vi "Query Octree with sphere.vi"(2 "Octree node array":T2[](array[typedef]), 3 "Sphere":T1) -> (0 "Stack error":errorcluster, 1 "Indices of possible triangles":i32[](array[numeric]))   [LabVIEW 2014]
uses:
  Typedefs/TreeNodeBox.ctl
  Typedefs/Quad.ctl
  Typedefs/Sphere.ctl
panel:
  out "Stack history":i32(graph)
  # "PN 18/01/2015"
  # "Vertices"
  # "Edges"
  # "Unit normal"
  # "Edge unit normals"
  # "Vertices"
  # "Edges"
  # "Unit normal"
  # "Edge unit normals"
  # "Vertices"
  # "Edges"
  # "Unit normal"
  # "Edge unit normals"
  # "Vertices"
  # "Edges"
  # "Unit normal"
  # "Edge unit normals"
  # "Vertices"
  # "Edges"
  # "Unit normal"
  # "Edge unit normals"
  # "Vertices"
  # "Edges"
  # "Unit normal"
  # "Edge unit normals"
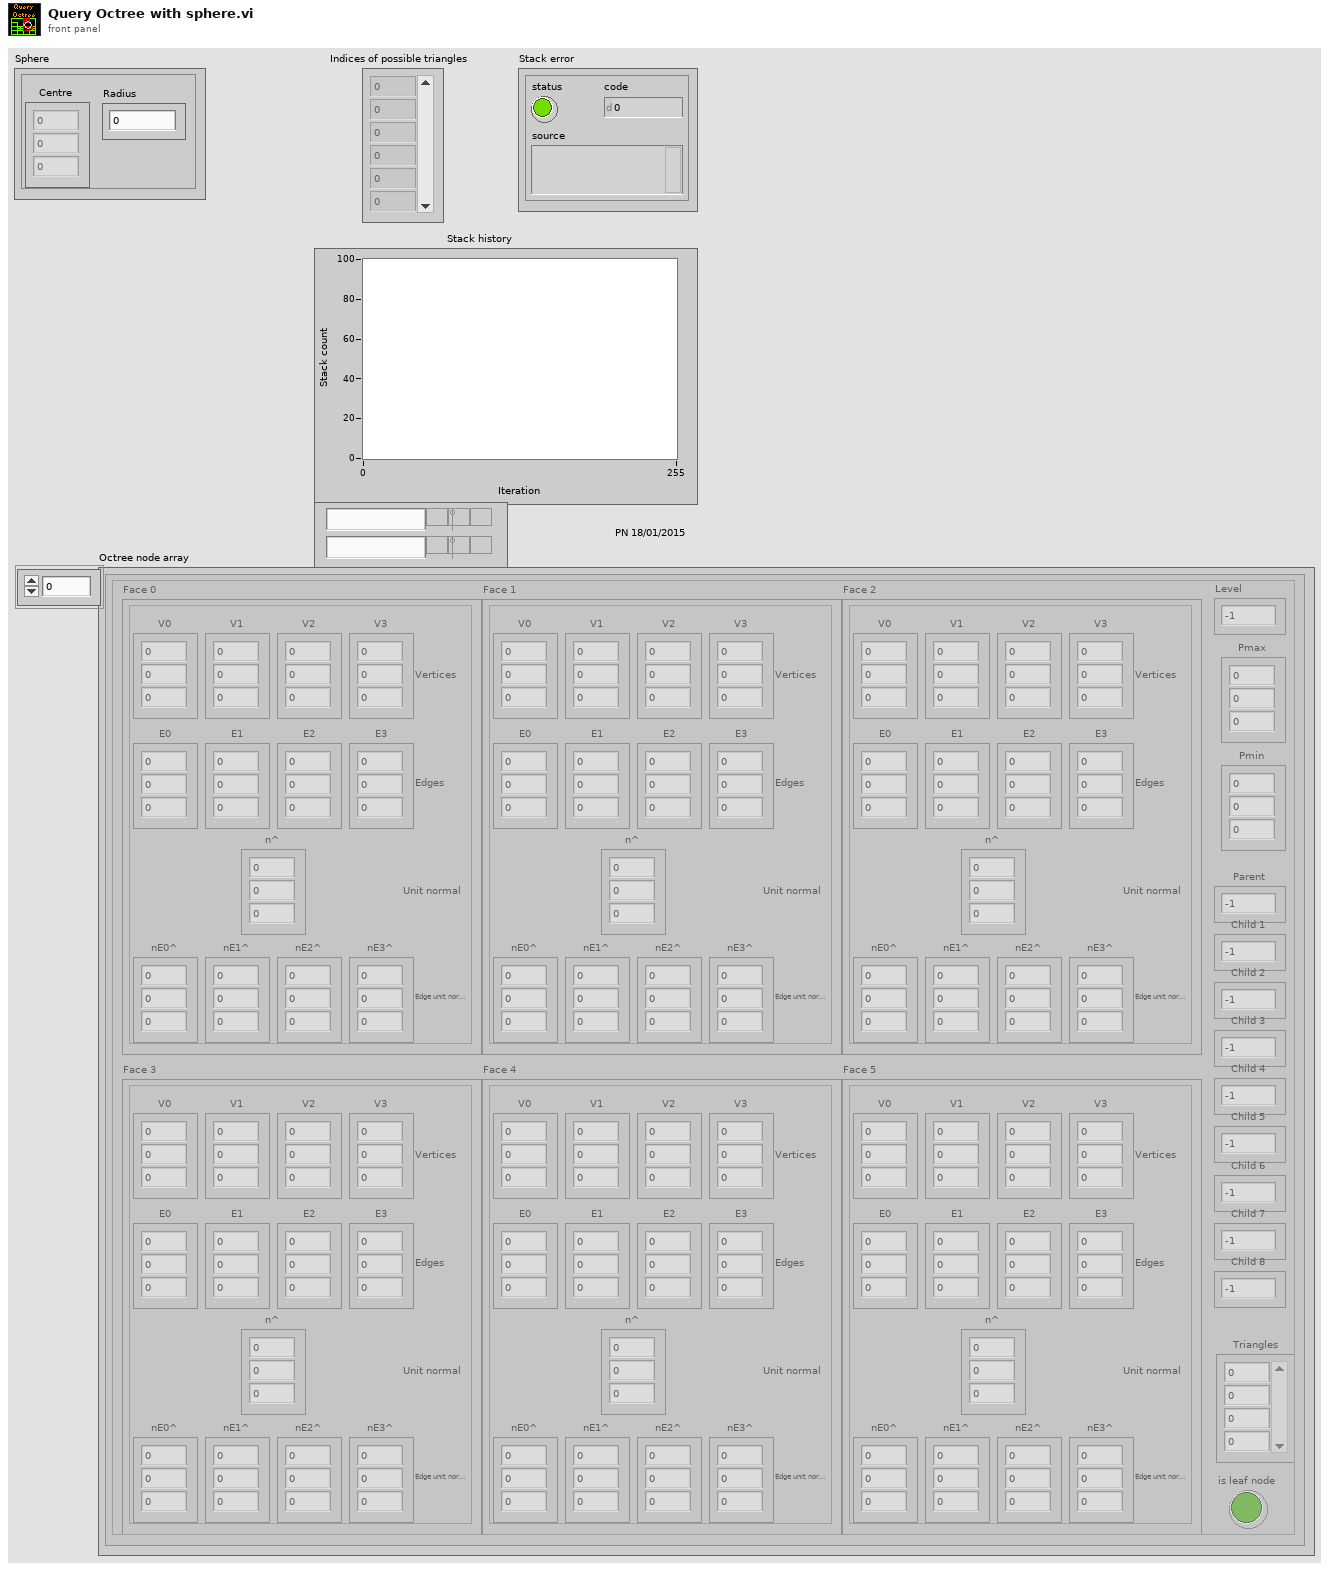
[diagram p1: front panel]
types:
  T1 = typedef "Sphere.ctl" = cluster{"Centre":sgl[], "Radius":sgl}
  T2 = typedef "TreeNodeBox.ctl" = cluster{"Face 0":T3, "Face 1":T3, "Face 2":T3, "Face 3":T3, "Face 4":T3, "Face 5":T3, "Level":i32, "Pmax":sgl[], "Pmin":sgl[], "Parent":i32, "Child 1":i32, "Child 2":i32, "Child 3":i32, "Child 4":i32, "Child 5":i32, "Child 6":i32, "Child 7":i32, "Child 8":i32, "Triangles":i32[], "is leaf node":bool}
  T3 = typedef "Quad.ctl" = cluster{"V0":sgl[], "V1":sgl[], "V2":sgl[], "V3":sgl[], "E0":sgl[], "E1":sgl[], "E2":sgl[], "E3":sgl[], "n^":sgl[], "nE0^":sgl[], "nE1^":sgl[], "nE2^":sgl[], "nE3^":sgl[]}
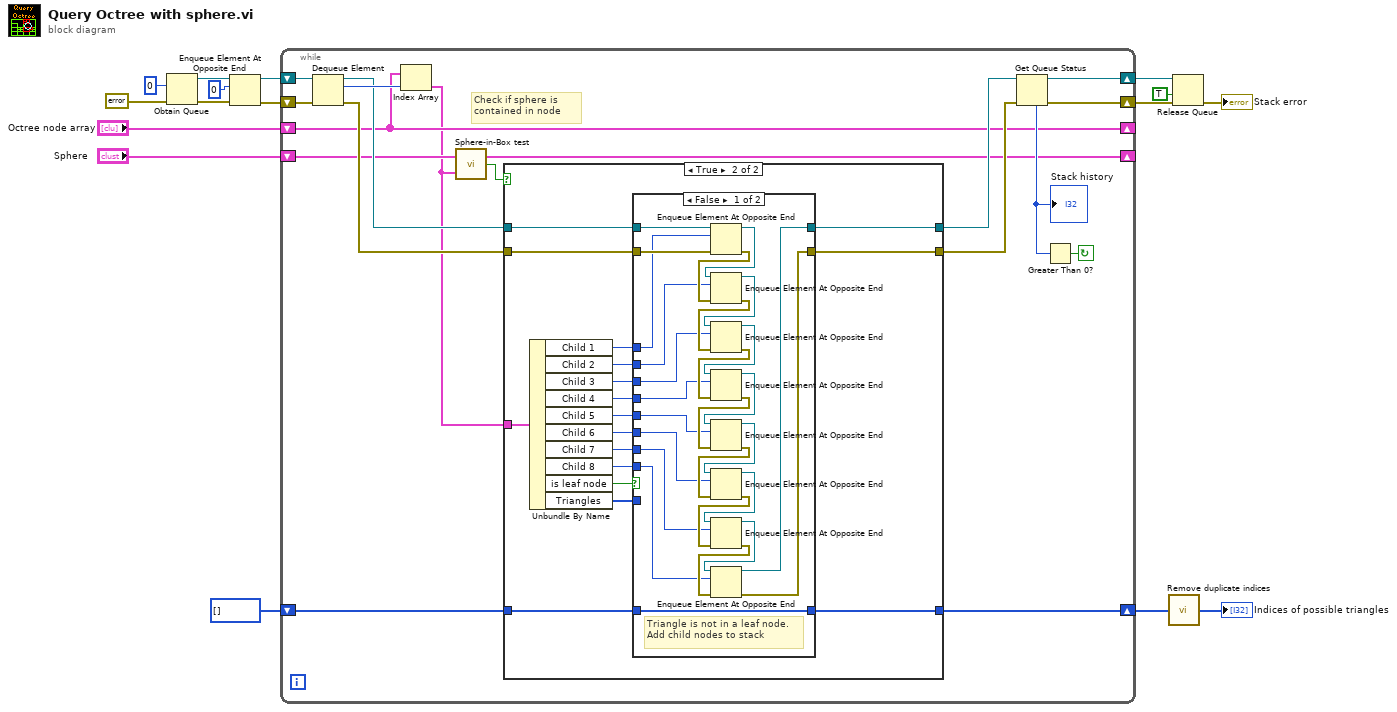
[diagram p0: block diagram]
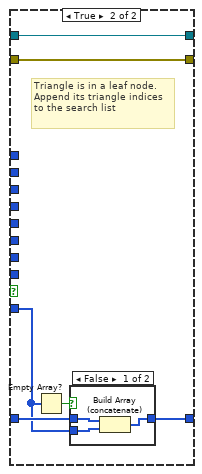
[diagram p3: hidden frame]
diagram:
  n1 = Obtain Queue(element data type=0, error in (no error)=errorcluster {"status"=FALSE, "code"=0, "source"=""}) -> (queue out=w15:refnum<queue>, error out=w14:errorcluster)  [unwired: 3 in, 1 out]
  n2 = Enqueue Element At Opposite End(queue=w15, element=0, error in (no error)=w14) -> (queue out=w13:refnum<queue>, error out=w12:errorcluster)  [unwired: 1 in, 1 out]
  n3 = while {
    shift-right: [w28] -> w11
    shift-left: w13 -> [w33]
    shift-right: [w30] -> w10
    shift-left: w12 -> [w32]
    shift-right: [w21] -> _
    shift-left: "Sphere" -> [w21]
    shift-right: [w20] -> _
    shift-left: "Octree node array" -> [w20]
    shift-right: [w17] -> w3
    shift-left: i32[] [] -> [w18]
    stop <- w31 continue-if-true
    # "Check if sphere is contained in node"
    n4 = Dequeue Element(queue=w33, error in (no error)=w32) -> (queue out=w27:refnum<queue>, element=w29:i32, error out=w26:errorcluster)  [unwired: 1 in, 1 out]
    n5 = Index Array(array=w20, index=w29) -> (element=w19:T2)
    n6 = call "Sphere-in-Box test.vi"("Box"=w19, "Sphere"=w21) -> ("Sphere is inside box"=w22:bool)
    n7 = case shown="True" w22 {
      tunnel: w27 -> [w35 w42]
      tunnel: [w35 w38] -> w25
      tunnel: [w36 w37] -> w24
      tunnel: w26 -> [w36 w41]
      tunnel: w19 -> [_ w53]
      tunnel: w18 -> [w34 w52]
      tunnel: [w34 w51] -> w17
      frame False {
        # "Triangle is not contained in node, continue"
      }
      frame True {
        n8 = Unbundle By Name(w53) -> ("Child 1"=w50:i32, "Child 2"=w49:i32, "Child 3"=w48:i32, "Child 4"=w47:i32, "Child 5"=w46:i32, "Child 6"=w45:i32, "Child 7"=w44:i32, "Child 8"=w43:i32, "is leaf node"=w40:bool, "Triangles"=w39:i32[])
        n9 = case shown="False" w40 {
          tunnel: w52 -> [w54 w85]
          tunnel: [w54 w84] -> w51
          tunnel: w50 -> [w64 _]
          tunnel: w49 -> [w63 _]
          tunnel: w48 -> [w62 _]
          tunnel: w47 -> [w61 _]
          tunnel: w46 -> [w60 _]
          tunnel: w45 -> [w59 _]
          tunnel: w44 -> [w58 _]
          tunnel: w43 -> [w57 _]
          tunnel: w39 -> [_ w83]
          tunnel: w42 -> [w66 w81]
          tunnel: w41 -> [w65 w82]
          tunnel: [w56 w81] -> w38
          tunnel: [w55 w82] -> w37
          frame False {
            # "Triangle is not in a leaf node.\nAdd child nodes to stack"
            n10 = Enqueue Element At Opposite End(queue=w66, element=w64, error in (no error)=w65) -> (queue out=w79:refnum<queue>, error out=w80:errorcluster)  [unwired: 1 in, 1 out]
            n11 = Enqueue Element At Opposite End(queue=w79, element=w63, error in (no error)=w80) -> (queue out=w78:refnum<queue>, error out=w77:errorcluster)  [unwired: 1 in, 1 out]
            n12 = Enqueue Element At Opposite End(queue=w78, element=w62, error in (no error)=w77) -> (queue out=w75:refnum<queue>, error out=w76:errorcluster)  [unwired: 1 in, 1 out]
            n13 = Enqueue Element At Opposite End(queue=w75, element=w61, error in (no error)=w76) -> (queue out=w73:refnum<queue>, error out=w74:errorcluster)  [unwired: 1 in, 1 out]
            n14 = Enqueue Element At Opposite End(queue=w73, element=w60, error in (no error)=w74) -> (queue out=w71:refnum<queue>, error out=w72:errorcluster)  [unwired: 1 in, 1 out]
            n15 = Enqueue Element At Opposite End(queue=w71, element=w59, error in (no error)=w72) -> (queue out=w69:refnum<queue>, error out=w70:errorcluster)  [unwired: 1 in, 1 out]
            n16 = Enqueue Element At Opposite End(queue=w69, element=w58, error in (no error)=w70) -> (queue out=w67:refnum<queue>, error out=w68:errorcluster)  [unwired: 1 in, 1 out]
            n17 = Enqueue Element At Opposite End(queue=w67, element=w57, error in (no error)=w68) -> (queue out=w56:refnum<queue>, error out=w55:errorcluster)  [unwired: 1 in, 1 out]
          }
          frame True {
            # "Triangle is in a leaf node.\nAppend its triangle indices to the search list"
            n18 = Empty Array?(array=w83) -> (empty?=w86:bool)
            n19 = case shown="False" w86 {
              tunnel: w83 -> [w89 _]
              tunnel: w85 -> [w88 w90]
              tunnel: [w87 w90] -> w84
              frame False {
                n20 = Build Array (concatenate)(w88, w89) -> (w87:i32[])
              }
              frame True {
              }
            }
          }
        }
      }
    }
    n21 = Get Queue Status(queue=w25, error in (no error)=w24) -> (queue out=w28:refnum<queue>, error out=w30:errorcluster, # elements in queue=w23:i32)  [unwired: 1 in, 5 out]
    "Stack history" <- w23
    n22 = Greater Than 0?(x=w23) -> (x > 0?=w31:bool)
  }
  n23 = call "Remove duplicate indices.vi"("I32 array with duplicates"=w3) -> ("I32 array without duplicates"=→"Indices of possible triangles":i32[])
  n24 = Release Queue(queue=w11, force destroy? (F)=TRUE, error in (no error)=w10) -> (error out=→"Stack error":errorcluster)  [unwired: 2 out]
